vi "Version Scripting.vi"(9 "Project":refnum<vi>, 10 "To":T1, 11 "From":T1) -> ()   [LabVIEW 2020]
uses:
  Version.ctl
  Tags.ctl
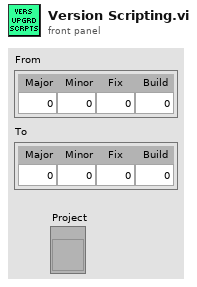
[diagram p1: front panel]
types:
  T1 = typedef "Version.ctl" = cluster{"Major":u16, "Minor":u16, "Fix":u16, "Build":u16}
  T2 = typedef "Tags.ctl" = enum16{"sol.squarebattle.version"}
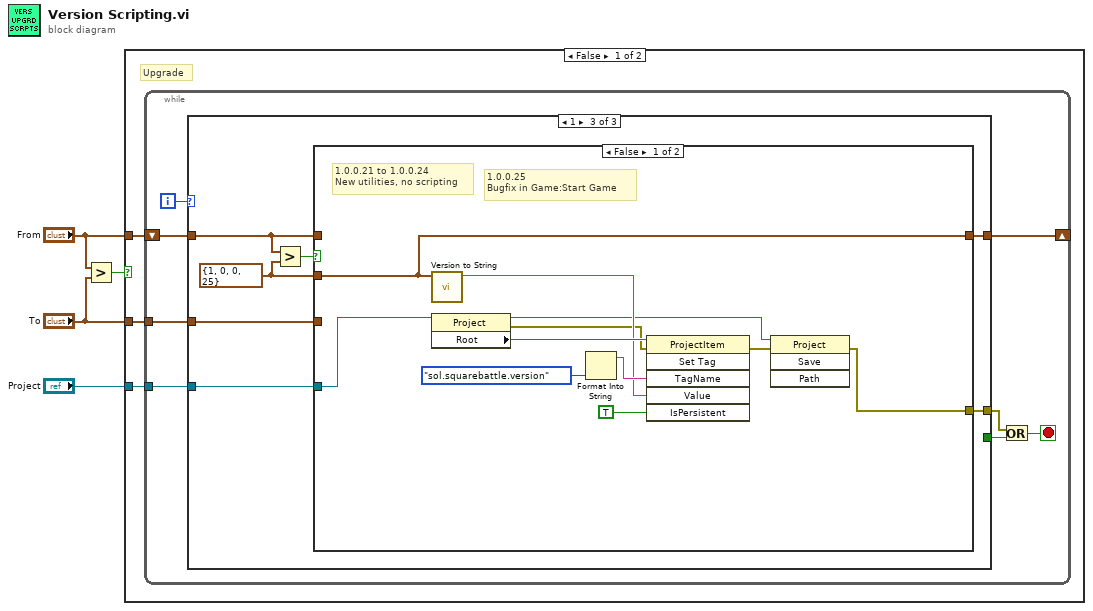
[diagram p0: block diagram]
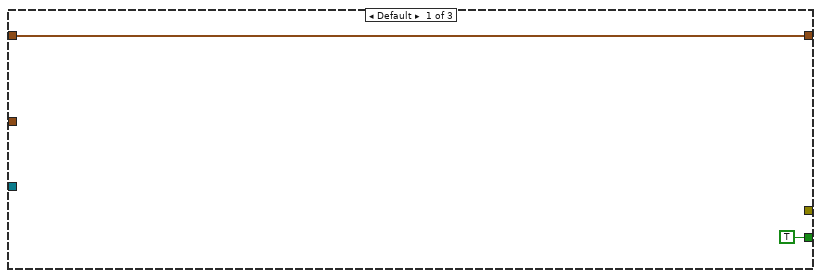
[diagram p2: hidden frame]
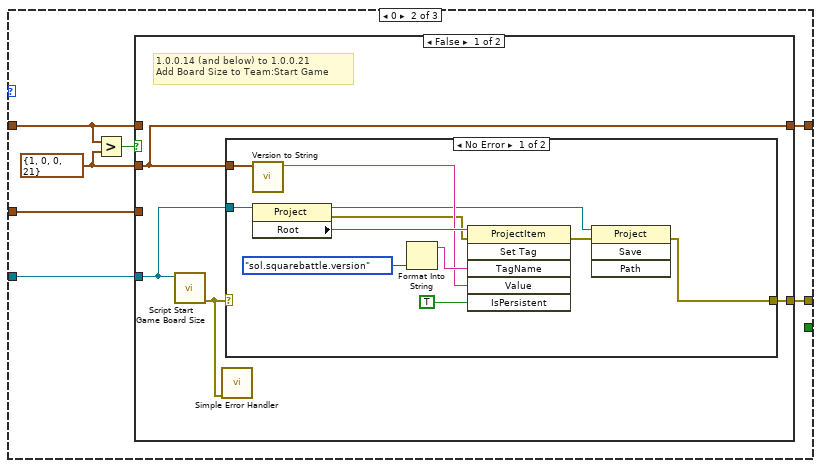
[diagram p3: hidden frame]
diagram:
  n1 = Greater?(x="From", y="To") -> (0:w1:bool)
  n2 = case shown="False" w1 {
    tunnel: "Project" -> [w7 _]
    tunnel: "From" -> [w6 _]
    tunnel: "To" -> [w5 _]
    frame False {
      # "Upgrade"
      n3 = while {
        shift-right: [w13] -> _
        shift-left: w6 -> [w14]
        tunnel: w7 -> [w10]
        tunnel: w5 -> [w12]
        i -> [w15]
        stop <- w9 stop-if-true
        n4 = case shown="1" w15 {
          tunnel: w14 -> [w16 w22 w46]
          tunnel: [w16 w21 w45] -> w13
          tunnel: w12 -> [_ w20 w44]
          tunnel: [TRUE _ _] -> w11
          tunnel: w10 -> [_ w19 w43]
          tunnel: [_ w18 w42] -> w8
          frame Default {
          }
          frame 0 {
            w23 = T1 {"Major"=1, "Minor"=0, "Fix"=0, "Build"=21} ("y")
            n5 = Greater?(x=w22, y=w23) -> (0:w24:bool)
            n6 = case shown="False" w24 {
              tunnel: w23 -> [w26 _]
              tunnel: w22 -> [_ w41]
              tunnel: [w26 w41] -> w21
              tunnel: w20 -> [_ _]
              tunnel: w19 -> [w27 _]
              tunnel: [w25 _] -> w18
              frame False {
                # "1.0.0.14 (and below) to 1.0.0.21\nAdd Board Size to Team:Start Game"
                n7 = call "Script Start Game Board Size.vi"("Project"=w27) -> ("error out"=w28:errorcluster)  [unwired: 10 in]
                n8 = call <vilib>:"Simple Error Handler.vi"("error in (no error)"=w28) -> ()  [unwired: 4 in, 5 out]
                n9 = case shown="No Error" w28 {
                  selector: w28 -> [_ w40]
                  tunnel: w27 -> [w39 _]
                  tunnel: w26 -> [w35 _]
                  tunnel: [w29 w40] -> w25
                  frame No Error {
                    n10 = call "Version to String.vi"("Version"=w35) -> ("Version String"=w34:string)  [unwired: 10 in]
                    n11 = property class="Project"(reference=w39) -> (reference out=w31:refnum<vi>, error out=w32:errorcluster, "Root"=w38:refnum<vi>)  [unwired: 1 in]
                    n12 = Format Into String(Tags."sol.squarebattle.version" ("Tags")) -> (resulting string=w36:string)  [unwired: 3 in, 1 out]
                    n13 = invoke class="ProjectItem" method="Set Tag"(reference=w38, error in=w32, "TagName"=w36, "Value"=w34, "IsPersistent"=TRUE ("Is Persistent (T)")) -> (error out=w30:errorcluster)  [unwired: 1 in, 5 out]
                    n14 = invoke class="Project" method="Save"(reference=w31, error in=w30) -> (error out=w29:errorcluster)  [unwired: 2 in, 3 out]
                  }
                  frame Error {
                  }
                }
              }
              frame True {
                # "Already greater than 1.0.0.15, nothing to do for this step."
              }
            }
          }
          frame 1 {
            w47 = T1 {"Major"=1, "Minor"=0, "Fix"=0, "Build"=25} ("y")
            n15 = Greater?(x=w46, y=w47) -> (0:w48:bool)
            n16 = case shown="False" w48 {
              tunnel: w47 -> [w58 _]
              tunnel: w46 -> [_ w60]
              tunnel: [w58 w60] -> w45
              tunnel: w44 -> [_ _]
              tunnel: w43 -> [w59 _]
              tunnel: [w57 _] -> w42
              frame False {
                # "1.0.0.25\nBugfix in Game:Start Game"
                # "1.0.0.21 to 1.0.0.24\nNew utilities, no scripting"
                n17 = call "Version to String.vi"("Version"=w58) -> ("Version String"=w53:string)  [unwired: 10 in]
                n18 = property class="Project"(reference=w59) -> (reference out=w50:refnum<vi>, error out=w51:errorcluster, "Root"=w56:refnum<vi>)  [unwired: 1 in]
                n19 = Format Into String(Tags."sol.squarebattle.version" ("Tags")) -> (resulting string=w54:string)  [unwired: 3 in, 1 out]
                n20 = invoke class="ProjectItem" method="Set Tag"(reference=w56, error in=w51, "TagName"=w54, "Value"=w53, "IsPersistent"=TRUE ("Is Persistent (T)")) -> (error out=w49:errorcluster)  [unwired: 1 in, 5 out]
                n21 = invoke class="Project" method="Save"(reference=w50, error in=w49) -> (error out=w57:errorcluster)  [unwired: 2 in, 3 out]
              }
              frame True {
                # "Already greater than 1.0.0.15, nothing to do for this step."
              }
            }
          }
        }
        n22 = Or(x=w8, y=w11) -> (x .or. y?=w9:bool)
      }
    }
    frame True {
      # "Downgrade"
    }
  }
